vi "LabView360-6-2.vi"() -> ()   [LabVIEW 2017]
panel:
  in  "STOP":bool
  in  "ADD":bool
  in  "数值":dbl
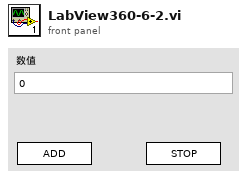
[diagram p1: front panel]
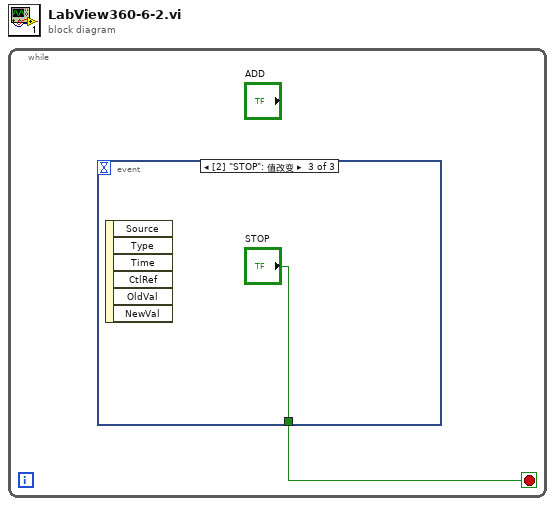
[diagram p0: block diagram]
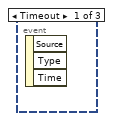
[diagram p2: hidden frame]
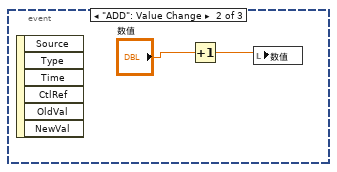
[diagram p3: hidden frame]
diagram:
  n1 = while {
    stop <- w1 stop-if-true
    n2 = event shown="[2] \"STOP\": 值改变" {
      selector: _ -> [_ _ _]
      dyn-events: _ -> [_ _ _]
      timeout: _ -> [_ _ _]
      tunnel: [_ _ "STOP"] -> w1
      event Timeout {
        n3 = event-data() -> ()  [unwired: 1 in, 3 out]
      }
      event "ADD": Value Change {
        n4 = event-data() -> ()  [unwired: 1 in, 6 out]
        n5 = Increment(x="数值") -> (x+1=w2:dbl)
        n6 = local write "数值"(w2) -> ()
      }
      event "STOP": Value Change {
        n7 = event-data() -> ()  [unwired: 1 in, 6 out]
      }
    }
  }
